vi "Acquire_nodt.vi"(0 "Ch Armed Reg":refnum<k21>="Register 1", 1 "Command FIFO":refnum<k21>, 3 "Circular Buffer Mem":refnum<k21>, 4 "circular buffer length":u32=300, 5 "FPGA I/O In":refnum<k21>="IO Module\\AI A0", 7 "channel on/off":bool, 9 "Trigger":i16=1500, 10 "Timing FIFO":refnum<k21>, 11 "Samples to Acquire":u32=100, 12 "Simulate":bool, 14 "# of pretrigger":u32=15, 15 "timing":u64) -> ()   [LabVIEW 2012]
uses:
  <vilib>/rvi/DataTransferAndStorage/Container/Common/niFpgaContainerExecOnDevCompGetState.vi
  <vilib>/rvi/Memory/Memory_Emulation/nirvimemoryEmulationManagerCache_GetValue.vi
  <vilib>/rvi/Memory/Memory_Emulation/niFpgaMemoryEmulationValidateCache.vi
  <vilib>/rvi/DataTransferAndStorage/Container/Common/niFpgaContainerGetUniqueNameForEmu.vi
  <vilib>/rvi/Memory/Memory_Emulation/nirvimemoryEmulationManagerCache_InsertValue.vi
  <vilib>/rvi/eio/common/nirviEmuTemplateMethod_errors.vi
  <vilib>/rvi/Emulation/niFpgaSctlEmulationGetInTimedLoop.vi
  <vilib>/rvi/FIFO/Fifo_Resource/nirvififoEmulationSetSize.vi
  <vilib>/rvi/errors/niFpgaSetErrorForExecOnDevCompSimple.vi
  <vilib>/rvi/eio/common/nirviEmuReportErrorAndStop.vi
  <vilib>/rvi/Emulation/niFpgaSctlEmulationFifoFullMgr.vi
  <vilib>/rvi/Emulation/niFpgaSctlEmulationResourceMgr.vi
  <vilib>/rvi/interface/RandomDataEmulation/nirviRandomDataFPGAFIFO.vi
  <vilib>/rvi/interface/RandomDataEmulation/niFpgaRandomDataHandleErrors.vi
  <vilib>/rvi/DataTransferAndStorage/Container/XNode/niFpgaContainer.xnode
  <vilib>/rvi/DataTransferAndStorage/Register/Emulation/niFpgaRegisterEmulationRefIn.vi
  <vilib>/eio/EIONode/EIONode.xnode
  <vilib>/rvi/FIFO/Fifo_Resource/niFpgaFifoEmulationRefIn.vi
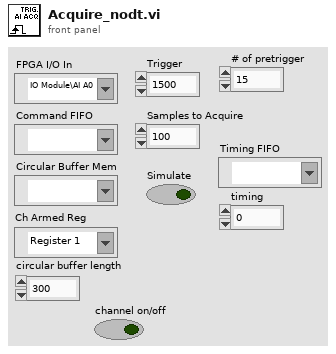
[diagram p1: front panel]
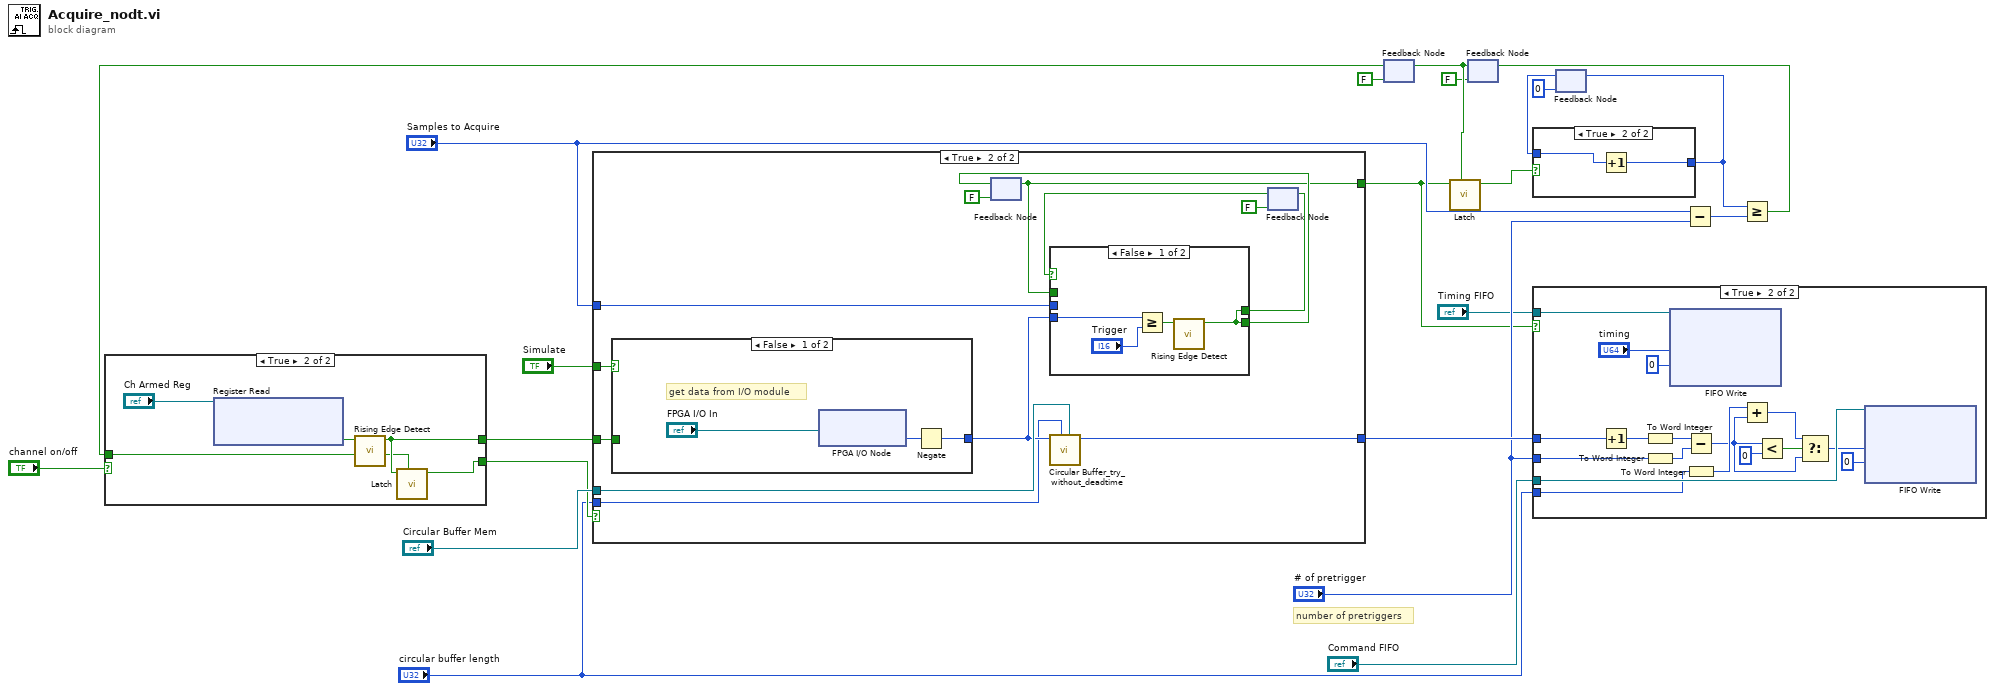
[diagram p0: block diagram]
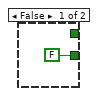
[diagram p2: hidden frame]
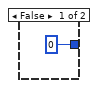
[diagram p3: hidden frame]
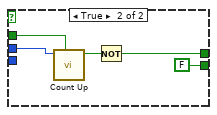
[diagram p5: hidden frame]
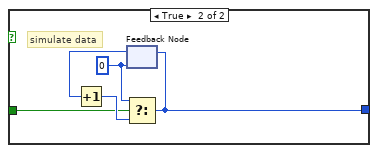
[diagram p6: hidden frame]
diagram:
  # "number of pretriggers"
  n1 = feedback #1(FALSE ("Count Met")) -> (w12:bool)
  n2 = case shown="True" "channel on/off" {
    tunnel: [FALSE ("Output") w26] -> w19
    tunnel: [_ w25] -> w18
    tunnel: w12 -> [_ w24]
    frame False {
    }
    frame True {
      n3 = xnode ("Register Read")("Register In"="Ch Armed Reg") -> ("Data"=w27:bool)  [unwired: 1 out]
      n4 = call "Rising Edge Detect.vi"("Input"=w27) -> ("Rising Edge"=w25:bool)  [unwired: 10 in]
      n5 = call "Latch.vi"("Reset"=w24, "Input"=w25) -> ("Output"=w26:bool)  [unwired: 9 in]
    }
  }
  n6 = case shown="True" w19 {
    tunnel: "Circular Buffer Mem" -> [_ w41]
    tunnel: "circular buffer length" -> [_ w39]
    tunnel: [_ w38] -> w20
    tunnel: w18 -> [_ w37]
    tunnel: "Simulate" -> [_ w36]
    tunnel: "Samples to Acquire" -> [_ w32]
    tunnel: [_ w30] -> w1
    frame False {
    }
    frame True {
      n7 = case shown="False" w36 {
        tunnel: [w51 w55] -> w40
        tunnel: w37 -> [_ w54]
        frame False {
          # "get data from I/O module"
          n8 = xnode "FPGA I/O Node"("FPGA I/O In"="FPGA I/O In") -> ("I/O Item"=w53:i16)  [unwired: 1 out]
          n9 = Negate(x=w53) -> (-x=w51:i16)
        }
        frame True {
          w56 = i16 0 ("x")
          # "simulate data"
          n10 = feedback #2(w56) -> (w58:i16)
          n11 = Increment(x=w58) -> (x+1=w57:i16)
          n12 = Select(t=w56, s=w54, f=w57) -> (s? t:f=w55:i16)
          n13 = feedback-in #2(w55) -> ()
        }
      }
      n14 = feedback #3(FALSE ("Rising Edge")) -> (w30:bool)
      n15 = call "Circular Buffer_try_without_deadtime.vi"("Refnum in"=w41, "circular buffer length"=w39, "Data"=w40) -> ("Address"=w38:u16)  [unwired: 8 in]
      n16 = feedback #4(FALSE ("Rising Edge")) -> (w35:bool)
      n17 = case shown="False" w35 {
        tunnel: w40 -> [w45 _]
        tunnel: [w42 w48] -> w33
        tunnel: w32 -> [_ w50]
        tunnel: [w42 FALSE ("Rising Edge")] -> w31
        tunnel: w30 -> [_ w47]
        frame False {
          n18 = Greater Or Equal?(x=w45, y="Trigger") -> (x >= y?=w43:bool)
          n19 = call "Rising Edge Detect.vi"("Input"=w43) -> ("Rising Edge"=w42:bool)  [unwired: 10 in]
        }
        frame True {
          n20 = call "Count Up.vi"("Reset?"=w47, "goal"=w50) -> ("Count Met"=w49:bool)  [unwired: 8 in, 1 out]
          n21 = Not(x=w49) -> (.not. x?=w48:bool)
        }
      }
      n22 = feedback-in #3(w31) -> ()
      n23 = feedback-in #4(w33) -> ()
    }
  }
  n24 = feedback #5(FALSE) -> (w14:bool)
  n25 = feedback-in #1(w14) -> ()
  n26 = call "Latch.vi"("Reset"=w14, "Input"=w1) -> ("Output"=w11:bool)  [unwired: 9 in]
  n27 = case shown="True" w1 {
    tunnel: "Command FIFO" -> [_ w75]
    tunnel: w20 -> [_ w60]
    tunnel: "# of pretrigger" -> [_ w61]
    tunnel: "circular buffer length" -> [_ w59]
    tunnel: "Timing FIFO" -> [_ w73]
    frame False {
    }
    frame True {
      n28 = Increment(x=w60) -> (x+1=w68:u16)
      n29 = To Word Integer(number=w68) -> (16bit integer=w69:i16)
      n30 = To Word Integer(number=w61) -> (16bit integer=w70:i16)
      n31 = xnode ("FIFO Write")("Element"="timing", "Timeout"=0, "FIFO In"=w73) -> ()  [unwired: 2 out]
      n32 = Subtract(x=w69, y=w70) -> (x-y=w66:i16)
      n33 = To Word Integer(number=w59) -> (16bit integer=w67:i16)
      n34 = Add(x=w67, y=w66) -> (x+y=w65:i16)
      n35 = Less?(x=w66, y=i16 0) -> (x < y?=w63:bool)
      n36 = Select(t=w65, s=w63, f=w66) -> (s? t:f=w62:i16)
      n37 = xnode ("FIFO Write")("Element"=w62, "Timeout"=0, "FIFO In"=w75) -> ()  [unwired: 2 out]
    }
  }
  n38 = feedback #6(u32 0) -> (w7:u32)
  n39 = case shown="True" w11 {
    tunnel: [u32 0 w78] -> w5
    tunnel: w7 -> [_ w77]
    frame False {
    }
    frame True {
      n40 = Increment(x=w77) -> (x+1=w78:u32)
    }
  }
  n41 = feedback-in #6(w5) -> ()
  n42 = Subtract(x="Samples to Acquire", y="# of pretrigger") -> (x-y=w10:u32)
  n43 = Greater Or Equal?(x=w5, y=w10) -> (x >= y?=w9:bool)
  n44 = feedback-in #5(w9) -> ()
